vi "LVFunction_Imop_SlopesPostProcessor_Apply Double Path.vi"(0 "HasoSlopes in":refnum<class "HasoSlopes.lvclass">, 5 "HasoSlopes OUT":refnum<class "HasoSlopes.lvclass">, 7 "doublePath":T1, 11 "error in (no error)":errorcluster) -> (4 "HasoSlopes out":refnum<class "HasoSlopes.lvclass">, 6 "HasoSlopes OUT 2":refnum<class "HasoSlopes.lvclass">, 15 "error out":errorcluster)   [LabVIEW 2020]
doc: "Divides the HasoSlopes by two.May ignore tilt and / or curvature depending on\nparametrization.\n\n<B>Slopes_inIn</B> : HasoSlopes object, modified by the processor if Slopes_out = NULL.\n<B>Slopes_inOut</B> : HasoSlopes object, modified by the processor if Slopes_out = NULL.\n<B>is_doublePath_active_on_tilt</B> : Is Double path active on tilt.\n<B>is_doublePath_active_on_curv</B> : Is Double path is active on curvature.\n<B>Slopes_out</B> : processed HasoSlopes object if not NULL."
uses:
  Classes/HasoSlopes/HasoSlopes.lvclass
  Controls/SlopesPostProcessorList - Double passage.ctl
  Classes/HasoSlopes/LVClass_HasoSlopes Read HasoSlopes _ property.vi
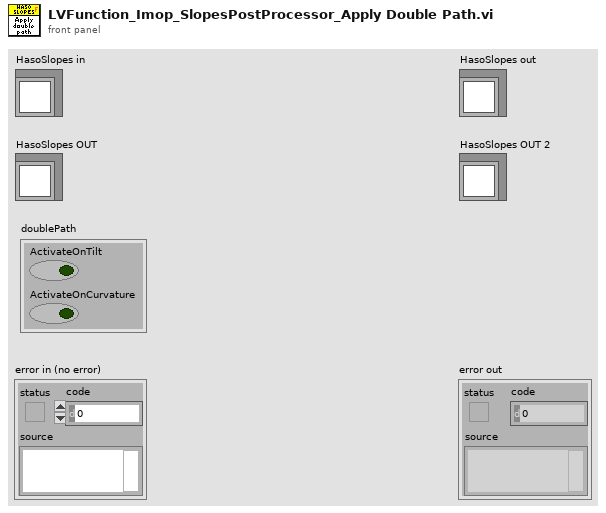
[diagram p1: front panel]
types:
  T1 = typedef "SlopesPostProcessorList - Double passage.ctl" = cluster{"ActivateOnTilt":bool, "ActivateOnCurvature":bool}
  T2 = typedef "ClassID.ctl" = i64
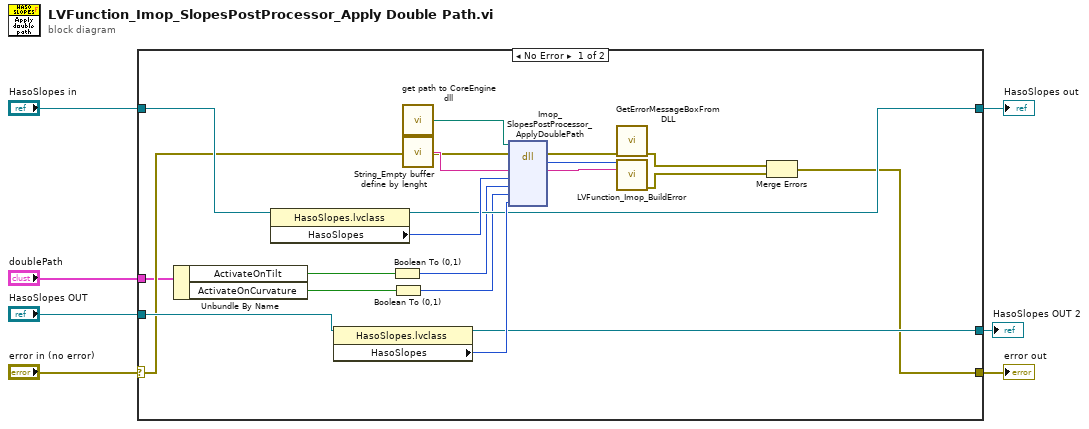
[diagram p0: block diagram]
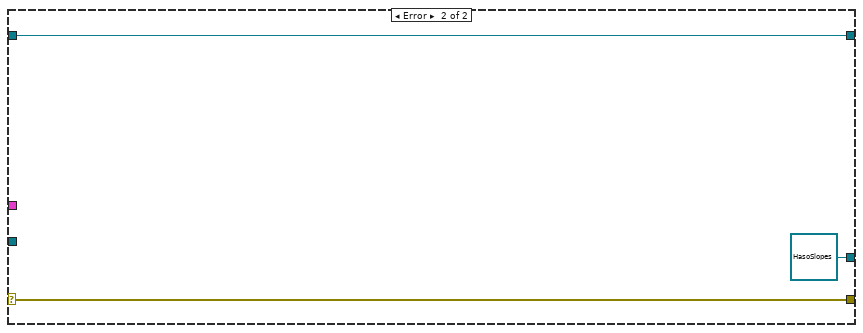
[diagram p2: hidden frame]
diagram:
  n1 = case shown="No Error" "error in (no error)" {
    selector: "error in (no error)" -> [w14 w30]
    tunnel: [w13 w30] -> w6
    tunnel: [w16 w29] -> w4
    tunnel: "HasoSlopes in" -> [w17 w29]
    tunnel: "HasoSlopes OUT" -> [w18 _]
    tunnel: [w15 refnum<class "HasoSlopes.lvclass"> refnum ("HasoSlopes OUT")] -> w2
    tunnel: "doublePath" -> [w11 _]
    frame No Error {
      n2 = Unbundle By Name(w11) -> ("ActivateOnTilt"=w9:bool, "ActivateOnCurvature"=w10:bool)
      n3 = property class="HasoSlopes.lvclass"(reference=w17) -> (reference out=w16:refnum<class "HasoSlopes.lvclass">, "HasoSlopes"=w27:T2)  [unwired: 1 in, 1 out]
      n4 = property class="HasoSlopes.lvclass"(reference=w18) -> (reference out=w15:refnum<class "HasoSlopes.lvclass">, "HasoSlopes"=w19:T2)  [unwired: 1 in, 1 out]
      n5 = Boolean To (0,1)(Boolean=w9) -> (0, 1=w8:i16)
      n6 = Boolean To (0,1)(Boolean=w10) -> (0, 1=w12:i16)
      n7 = call "get path to CoreEngine dll.vi"() -> ("path to wavekit library"=w22:path)  [unwired: 14 in, 1 out]
      n8 = call "String_Empty buffer define by lenght.vi"() -> ("Empty buffer"=w23:string)  [unwired: 1 in]
      n9 = dll-call lib="D:/FLE/0.Code/CoreEngine4_Suite/LV2011_interface/DLLs/c_interface_vc100.dll" fn="Imop_SlopesPostProcessor_ApplyDoublePath"(path in=w22, error in=w14, "Message"=w23, "HasoSlopes IN"=w27, "Double path on tilt"=w8, "Double path on curvature"=w12, "HasoSlopes OUT"=w19) -> (error out=w26:errorcluster, "return type"=w24:i32, "Message"=w25:string)  [unwired: 5 in, 1 out]
      n10 = call "GetErrorMessageBoxFromDLL.vi"("error IN"=w26) -> ("error OUT"=w21:errorcluster)  [unwired: 10 in]
      n11 = call "LVFunction_Imop_BuildError.vi"("code"=w24, "String to Prepend to source (\"\")"=w25) -> ("error out"=w20:errorcluster)  [unwired: 13 in]
      n12 = Merge Errors(w21, w20) -> (w13:errorcluster)
    }
    frame Error {
    }
  }
  "error out" <- w6
  "HasoSlopes out" <- w4
  "HasoSlopes OUT 2" <- w2
